vi "MeasurementServer_CreateServer.vi"() -> (3 "gRPCid":T1)   [LabVIEW 2019, in "labview-grpc-measurement-server.lvlib"]
uses:
  labview-grpc-measurement-server.lvlib
  MeasurementServer_gRPCid.ctl
  home/lvuser/liblabview_measurement_server.so
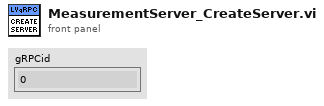
[diagram p1: front panel]
types:
  T1 = typedef "labview-grpc-measurement-server.lvlib/MeasurementServer_gRPCid.ctl" = u64
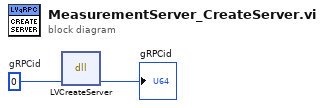
[diagram p0: block diagram]
diagram:
  w2 = T1 0  # gRPCid
  n1 = dll-call lib="home/lvuser/liblabview_measurement_server.so" fn="LVCreateServer"("server"=w2) -> ("server"=→"gRPCid":T1)  [unwired: 4 in, 2 out]
